vi "Error Query.vi"(8 "error in (no error)":errorcluster, 9 "Device and Axis":string, 11 "VISA resource name":refnum<visa-resource-name>) -> (0 "error out":errorcluster, 1 "Error Message":string, 2 "Error Code":i32, 3 "VISA resource name out":refnum<visa-resource-name>)   [LabVIEW 2012, in "Zaber A Series.lvlib"]
doc: "Queries the instrument for any warning flads. All warning flags will be returned in the order of descending severity. \n\nThis VI requires that the Initialize VI has been called with the same serial port."
uses:
  <instrlib>/Zaber A Series/Zaber A Series.lvlib
  <instrlib>/Zaber A Series/Private/All Commands.ctl
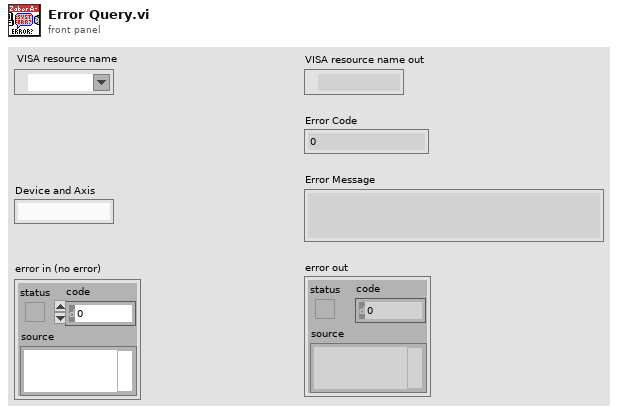
[diagram p1: front panel]
types:
  T1 = typedef "Zaber A Series.lvlib/All Commands.ctl" = string
  T2 = cluster{"Device":string, "Axis":string, "Reply Flag":string, "Status":string, "Warning Flags":string, "Data":string}[]
  T3 = cluster{"Device":string, "Axis":string, "Reply Flag":string, "Status":string, "Warning Flags":string, "Data":string}
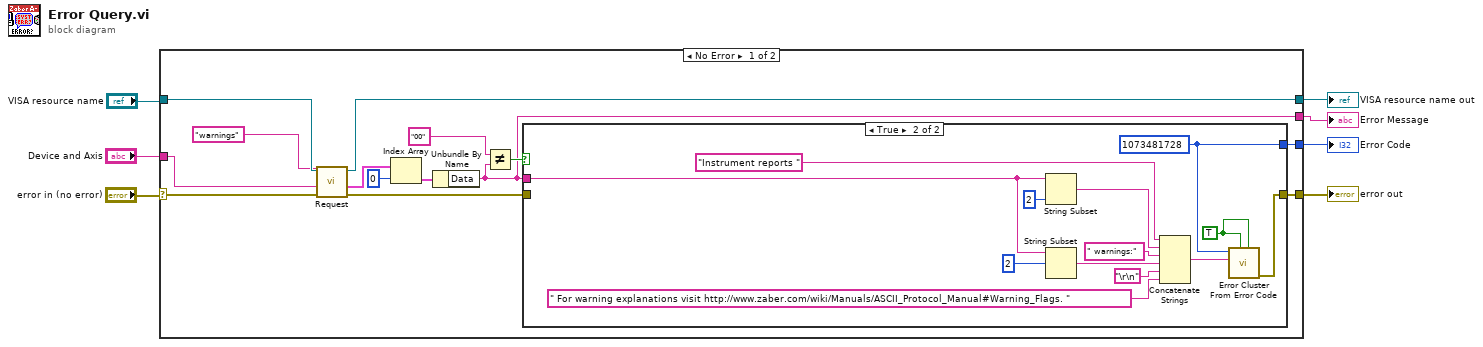
[diagram p0: block diagram]
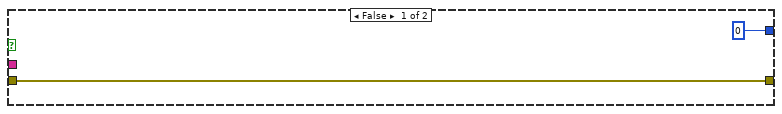
[diagram p2: hidden frame]
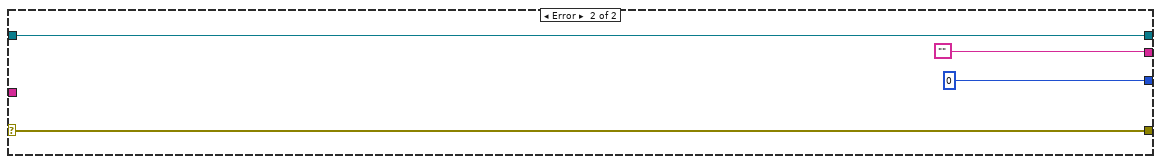
[diagram p3: hidden frame]
diagram:
  n1 = case shown="No Error" "error in (no error)" {
    selector: "error in (no error)" -> [w20 w39]
    tunnel: [w18 w40] -> w7
    tunnel: "VISA resource name" -> [w21 w40]
    tunnel: [w9 w39] -> w3
    tunnel: [w12 ""] -> w1
    tunnel: [w10 0 ("Code")] -> w4
    tunnel: "Device and Axis" -> [w8 _]
    frame No Error {
      n2 = call <instrlib>:"Request.vi"("error in (no error)"=w20, "Device and Axis"=w8, "Command String"=T1 "warnings" ("Warning Command"), "VISA resource name"=w21) -> ("error out"=w17:errorcluster, "Response Bundle Array"=w16:T2, "VISA resource name out"=w18:refnum<visa-resource-name>)  [unwired: 3 in, 2 out]
      n3 = Index Array(array=w16, index=0) -> (element=w14:T3)
      n4 = Unbundle By Name(w14) -> ("Data"=w12:string)
      n5 = Not Equal?(x="00" ("No Warning Data"), y=w12) -> (x != y?=w13:bool)
      n6 = case shown="True" w13 {
        tunnel: w12 -> [_ w24]
        tunnel: [w23 w34] -> w9
        tunnel: w17 -> [w23 _]
        tunnel: [0 ("Code") w25] -> w10
        frame False {
        }
        frame True {
          w33 = TRUE ("show call chain? (False)")
          w25 = 1073481728 ("Code")
          n7 = String Subset(string=w24, length (rest)=2 ("length (rest)")) -> (substring=w32:string)  [unwired: 1 in]
          n8 = String Subset(string=w24, offset (0)=2) -> (substring=w28:string)  [unwired: 1 in]
          n9 = Concatenate Strings("Instrument reports " ("Source"), w32, " warnings:" ("Source"), w28, "\r\n", " For warning explanations visit http://www.zaber.com/wiki/Manuals/ASCII_Protocol_Manual#Warning_Flags. " ("string")) -> (w35:string)
          n10 = call <vilib>:"Error Cluster From Error Code.vi"("is warning? (False)"=w33, "show call chain? (False)"=w33, "error message (\"\")"=w35, "error code (0)"=w25) -> ("error out"=w34:errorcluster)  [unwired: 5 in]
        }
      }
    }
    frame Error {
    }
  }
  "VISA resource name out" <- w7
  "Error Message" <- w1
  "Error Code" <- w4
  "error out" <- w3
